vi "PE Set Wavelength.vi"(8 "error in (no error)":errorcluster, 10 "wavelength":dbl, 11 "peHandle":u32) -> (0 "error out":errorcluster, 3 "function return":i32)   [LabVIEW 2011, in "libPhyspec.lvlib"]
doc: "PHYSPEC_API PE_STATUS PE_SetWavelength(PE_HANDLE peHandle, double wavelength);"
uses:
  libPhyspec.lvlib
  libPhyspec.dll
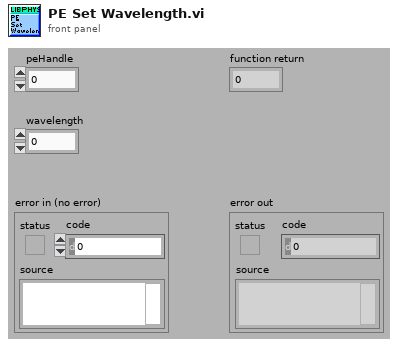
[diagram p1: front panel]
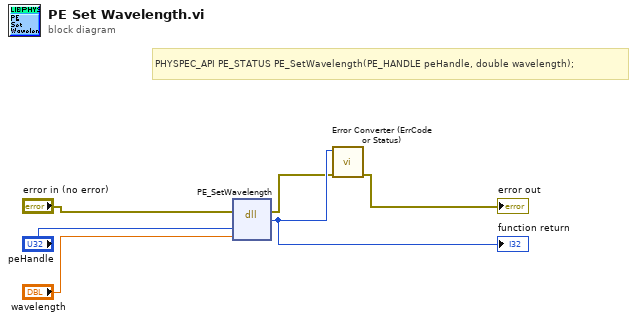
[diagram p0: block diagram]
diagram:
  # "PHYSPEC_API PE_STATUS PE_SetWavelength(PE_HANDLE peHandle, double wavelength);"
  n1 = dll-call lib="D:/users/nicolas/PHySpec-SDK-1.0.0/Labview-example/libPhyspec/libPhyspec.*" fn="PE_SetWavelength"(error in="error in (no error)", "peHandle"="peHandle", "wavelength"="wavelength") -> (error out=w2:errorcluster, w6:i32)  [unwired: 4 in, 1 out]
  "function return" <- w6
  n2 = call "Error Converter (ErrCode or Status).vi"("error in (no error)"=w2, "error code"=w6) -> ("error out"=→"error out":errorcluster)  [unwired: 9 in]
